vi "getCameraParameters.vi"(10 "error in (no error)":errorcluster, 11 "IMAQdx Session":T1) -> (1 "errorCameraParsRequest":errorcluster, 2 "VendorNameModelName":string, 3 "IPAddress":string)   [LabVIEW 2021]
uses:
  <vilib>/userdefined/High Color/IMAQdx.ctl
  <resource>/objmgr/imaqdx.rc
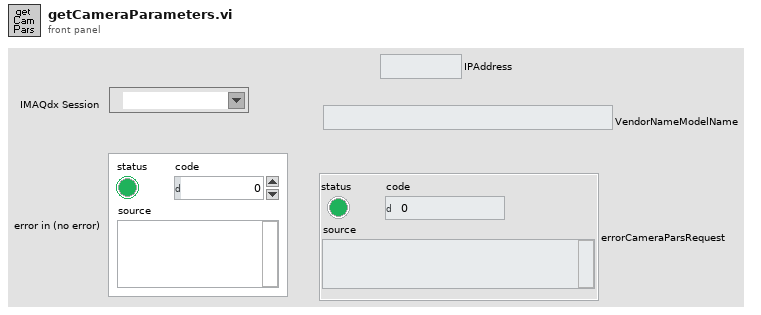
[diagram p1: front panel]
types:
  T1 = typedef "IMAQdx.ctl" = refnum<k21>
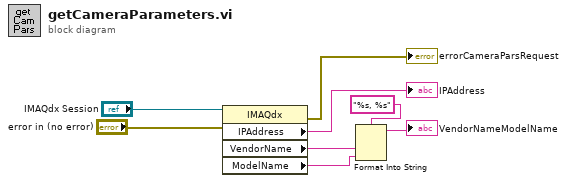
[diagram p0: block diagram]
diagram:
  n1 = property class="IMAQdx"(reference="IMAQdx Session", error in="error in (no error)") -> (error out=→"errorCameraParsRequest":errorcluster, "IPAddress"=→"IPAddress":string, "VendorName"=w4:string, "ModelName"=w5:string)  [unwired: 1 out]
  n2 = Format Into String(format string="%s, %s", w4, w5) -> (resulting string=→"VendorNameModelName":string)  [unwired: 2 in, 1 out]
